vi "Write States.vi"(8 "error in (no error)":errorcluster, 10 "States":enum16{"Exit", "Timeout"}(ring), 11 "TimeoutTactic in":refnum<class "TimeoutTactic.lvclass">) -> (0 "error out":errorcluster, 3 "TimeoutTactic out":refnum<class "TimeoutTactic.lvclass">)   [LabVIEW 2023, in "TimeoutTactic.lvclass"]
uses:
  TimeoutTactic.lvclass
  TimeoutTactic.lvclass/TimeoutTactic.ctl
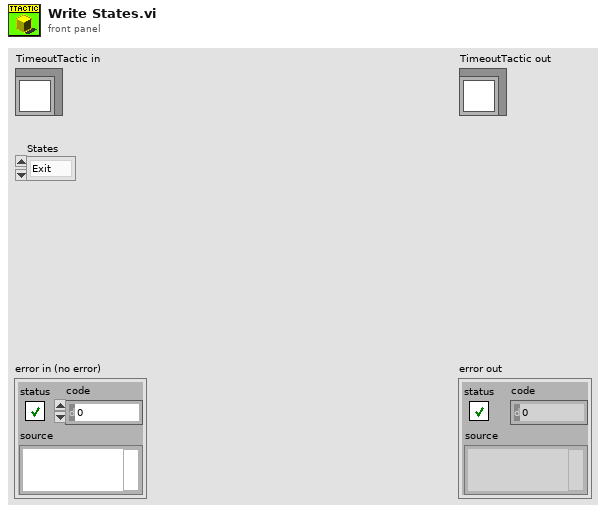
[diagram p1: front panel]
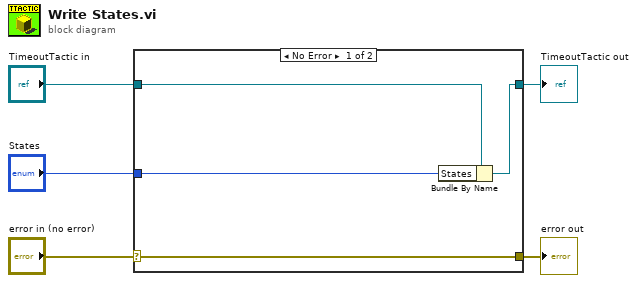
[diagram p0: block diagram]
diagram:
  n1 = case shown="No Error" "error in (no error)" {
    selector: "error in (no error)" -> [w9 w10]
    tunnel: [w9 w10] -> w4
    tunnel: [w7 w11] -> w2
    tunnel: "TimeoutTactic in" -> [w8 w11]
    tunnel: "States" -> [w6 _]
    frame No Error {
      n2 = Bundle By Name(cluster=w8, "States"=w6) -> (w7:refnum<class "TimeoutTactic.lvclass">)
    }
    frame Error {
    }
  }
  "error out" <- w4
  "TimeoutTactic out" <- w2
